vi "Switch_StoreInstrumentSession.vi"(8 "error in (no error)":errorcluster, 9 "Instrument Session":refnum<k15>, 10 "Instrument Name":string="dev1", 11 "Semiconductor Module Context":T1) -> (0 "error out":errorcluster, 3 "Semiconductor Module Context Out":T1)   [LabVIEW 2014]
uses:
  <vilib>/NI_TestStand_SemiconductorModule/NI_TestStand_Semiconductor_Module.lvlibp/PinMap/General/SemiconductorModuleContext.ctl
  <vilib>/NI_TestStand_SemiconductorModule/NI_TestStand_Semiconductor_Module.lvlibp
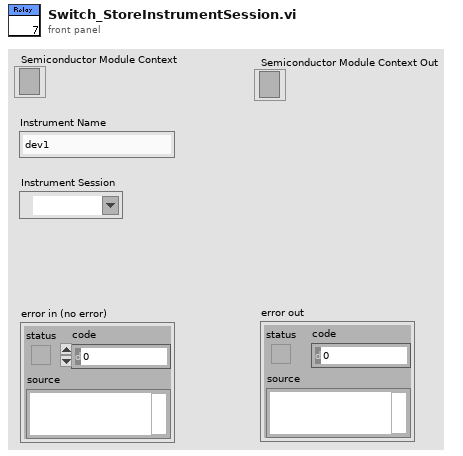
[diagram p1: front panel]
types:
  T1 = typedef "NI_TestStand_Semiconductor_Module.lvlibp/SemiconductorModuleContext.ctl" = refnum<k7>
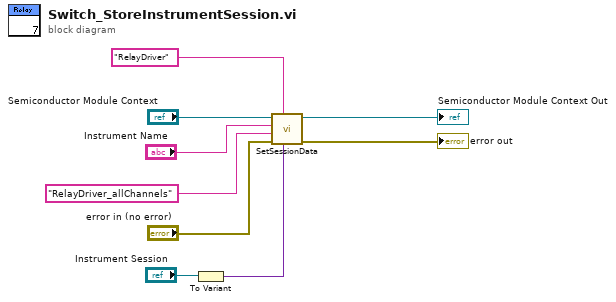
[diagram p0: block diagram]
diagram:
  n1 = To Variant(anything="Instrument Session") -> (Variant=w2:variant)
  n2 = call <vilib>:"SetSessionData.vi"("Session Data"=w2, "Instrument Type Id"="RelayDriver" ("Instrument Type"), "error in (no error)"="error in (no error)", "Channel Group Id"="RelayDriver_allChannels" ("channel group defined in pin map XML"), "Instrument Name"="Instrument Name", "Semiconductor Module Context"="Semiconductor Module Context") -> ("error out"=→"error out":errorcluster, "Semiconductor Module Context Out"=→"Semiconductor Module Context Out":T1)  [unwired: 4 in]
